vi "输入数据解析.vi"(0 "单个参数补充":dbl, 1 "从板号":dbl=1.0, 2 "主板二维码":string="BNET01", 3 "从板二维码":string="BNET01", 5 "主板引用":refnum<vi>, 7 "从板引用":refnum<vi>, 9 "主板选项":string="三级故障阀值", 11 "枚举":enum16{"主板", "从板"}(ring), 12 "快换":bool caption="快换写入") -> (4 "输出数组":dbl[][](array[numeric]), 6 "数组长度":dbl[](array[numeric]), 8 "循环次数":i32, 10 "命令":u32, 14 "名称":string[](array[string]), 15 "命令序号":u32[](array[numeric]))   [LabVIEW 2013] (continued)
                    n679 = call "输入分辨率计算-EV05.vi"("1字节?"=TRUE, "数值"=w1608, "偏移量"=0.0, "分辨率"=1.0) -> ("高字节1"=w1611:dbl)  [unwired: 1 in, 6 out]
                  }
                  frame Enabled {
                  }
                }
                n680 = Build Array(w1607) -> (w1606:i32[])
              }
              frame 12 {
                # "SOC过高"
                n681 = Unbundle By Name(w1619) -> ("SOC过高"=w1618:dbl)
                n682 = call "输入分辨率计算-EV05.vi"("1字节?"=FALSE, "数值"=w1618, "偏移量"=0.0, "分辨率"=0.1) -> ("低字节"=w1620:dbl, "高字节1"=w1621:dbl)  [unwired: 1 in, 5 out]
                n683 = call "二进制解析-8.6.vi"("索引"=4, "数值"=w1621) -> ("低位子数组"=w1624:i32[])  [unwired: 3 out]
                n684 = call "二进制解析-8.6.vi"("索引"=4, "数值"=w1620) -> ("低位子数组"=w1616:i32[], "高位子数组"=w1623:i32[])  [unwired: 2 out]
                n685 = Insert Into Array(array=w1624, new element=w1623) -> (w1622:i32[])  [unwired: 1 in]
                n686 = call "数值二进制转十进制-8.6.vi"("子数组"=w1622) -> ("十进制数值"=w1617:i32)  [unwired: 4 out]
                n687 = disable-structure shown="启用" {
                  disable-tunnel: w1617 -> [w1632 _]
                  disable-tunnel: [w1632 255 ("高字节1")] -> w1615
                  disable-tunnel: [w1631 i32[] [] ("低位子数组 20")] -> _
                  disable-tunnel: w1616 -> [w1631 _]
                  frame Disabled {
                  }
                  frame Enabled {
                  }
                }
                n688 = Build Array(w1615, w1615) -> (w1628:i32[])
              }
              frame 13 {
                # "SOC过低"
                n689 = Unbundle By Name(w1641) -> ("SOC过低"=w1640:dbl)
                n690 = call "输入分辨率计算-EV05.vi"("1字节?"=FALSE, "数值"=w1640, "偏移量"=0.0, "分辨率"=0.1) -> ("低字节"=w1638:dbl, "高字节1"=w1639:dbl)  [unwired: 1 in, 5 out]
                n691 = call "二进制解析-8.6.vi"("索引"=4, "数值"=w1639) -> ("低位子数组"=w1636:i32[])  [unwired: 3 out]
                n692 = disable-structure shown="启用" {
                  disable-tunnel: w1638 -> [w1648 _]
                  disable-tunnel: [w1648 255 ("高字节1")] -> w1637
                  disable-tunnel: w1636 -> [w1647 _]
                  disable-tunnel: [_ 255 ("高字节1")] -> w1635
                  frame Disabled {
                    (unwired) i32[] [] ("低位子数组 4")
                  }
                  frame Enabled {
                  }
                }
                n693 = Build Array(w1635, w1637) -> (w1644:i32[])
              }
              frame 14 {
                # "内阻过大"
                n694 = disable-structure shown="启用" {
                  disable-tunnel: w1653 -> [w1658 _]
                  disable-tunnel: [w1654 255 ("高字节1")] -> w1651
                  frame Disabled {
                    n695 = Unbundle By Name(w1658) -> ("内阻过大"=w1657:dbl)
                    n696 = call "输入分辨率计算-EV05.vi"("1字节?"=TRUE, "数值"=w1657, "分辨率"=0.1) -> ("高字节1"=w1654:dbl)  [unwired: 2 in, 6 out]
                  }
                  frame Enabled {
                  }
                }
                n697 = Build Array(w1651) -> (w1652:i32[])
              }
              frame 15 {
                # "极柱温度过高"
                n698 = disable-structure shown="启用" {
                  disable-tunnel: w1662 -> [w1668 _]
                  disable-tunnel: [w1664 255 ("高字节1")] -> w1660
                  frame Disabled {
                    n699 = Unbundle By Name(w1668) -> ("极柱温度过高"=w1667:dbl)
                    n700 = call "输入分辨率计算-EV05.vi"("1字节?"=TRUE, "数值"=w1667, "偏移量"=-40.0, "分辨率"=1.0) -> ("高字节1"=w1664:dbl)  [unwired: 1 in, 6 out]
                  }
                  frame Enabled {
                  }
                }
                n701 = Build Array(w1660) -> (w1661:i32[])
              }
              frame 16 {
                # "SOH过低"
                n702 = disable-structure shown="启用" {
                  disable-tunnel: [w1685 w1693] -> w1672
                  disable-tunnel: w1671 -> [w1682 _]
                  disable-tunnel: [w1674 w1693] -> w1670
                  frame Disabled {
                    n703 = Unbundle By Name(w1682) -> ("SOH过低"=w1681:dbl)
                    n704 = call "输入分辨率计算-EV05.vi"("1字节?"=FALSE, "数值"=w1681, "偏移量"=0.0, "分辨率"=0.1) -> ("低字节"=w1683:dbl, "高字节1"=w1684:dbl)  [unwired: 1 in, 5 out]
                    n705 = call "二进制解析-8.6.vi"("索引"=4, "数值"=w1684) -> ("低位子数组"=w1687:i32[])  [unwired: 3 out]
                    n706 = call "二进制解析-8.6.vi"("索引"=4, "数值"=w1683) -> ("低位子数组"=w1676:i32[], "高位子数组"=w1686:i32[])  [unwired: 2 out]
                    n707 = call "二进制解析-8.6.vi"("索引"=4, "数值"=0) -> ("低位子数组"=w1677:i32[])  [unwired: 3 out]
                    n708 = Insert Into Array(array=w1687, new element=w1686) -> (w1680:i32[])  [unwired: 1 in]
                    n709 = Insert Into Array(array=w1676, new element=w1677) -> (w1675:i32[])  [unwired: 1 in]
                    n710 = call "数值二进制转十进制-8.6.vi"("子数组"=w1680) -> ("十进制数值"=w1685:i32)  [unwired: 4 out]
                    n711 = call "数值二进制转十进制-8.6.vi"("子数组"=w1675) -> ("十进制数值"=w1674:i32)  [unwired: 4 out]
                  }
                  frame Enabled {
                    w1693 = 255 ("高字节1")
                  }
                }
                n712 = Build Array(w1672, w1670) -> (w1673:i32[])
              }
            }
            n713 = Insert Into Array(array=w1477, new element=w1478) -> (w1476:dbl[])  [unwired: 1 in]
          }
          n714 = Build Array(w1473) -> (w1472:dbl[][])
          n715 = Build Array("一级故障阀值") -> (w1463:string[])
        }
        frame "总电压过低(2)" {
          n716 = Unbundle By Name(w1699) -> ("一级故障 2"=w1700:refnum<vi>)
          n717 = property class="Clust (严格)"(reference=w1700) -> ("Value"=w1698:T4)  [unwired: 1 in, 2 out]
          n718 = for {
            N: 17 -> [_]
            tunnel: w1698 -> [w1710]
            shift-right: [w1707] -> w1704
            shift-left: dbl[] [] -> [w1708]
            i -> [w1711]
            n719 = case shown="13" w1711 {
              tunnel: w1710 -> [w1712 w1723 w1734 w1744 w1754 w1764 w1776 w1788 w1800 w1812 w1824 w1836 w1850 w1872 w1884 w1893 w1902]
              tunnel: [w1713 w1724 w1735 w1745 w1755 w1766 w1778 w1790 w1802 w1814 w1826 w1837 w1859 w1875 w1883 w1892 w1904] -> w1709
              frame 0, Default {
                # "总电压过高"
                n720 = disable-structure shown="启用" {
                  disable-tunnel: [w1719 w1722] -> w1715
                  disable-tunnel: [w1718 w1722] -> w1714
                  disable-tunnel: w1712 -> [w1717 _]
                  frame Disabled {
                    n721 = Unbundle By Name(w1717) -> ("总电压过高"=w1716:dbl)
                    n722 = call "输入分辨率计算-EV05.vi"("1字节?"=FALSE, "数值"=w1716, "分辨率"=0.1) -> ("低字节"=w1719:dbl, "高字节1"=w1718:dbl)  [unwired: 2 in, 5 out]
                  }
                  frame Enabled {
                    w1722 = 255 ("高字节1")
                  }
                }
                n723 = Build Array(w1714, w1715) -> (w1713:i32[])
              }
              frame 1 {
                # "总电压过低"
                n724 = disable-structure shown="启用" {
                  disable-tunnel: [w1730 w1733] -> w1726
                  disable-tunnel: [w1729 w1733] -> w1725
                  disable-tunnel: w1723 -> [w1728 _]
                  frame Enabled {
                    n725 = Unbundle By Name(w1728) -> ("总电压过低"=w1727:dbl)
                    n726 = call "输入分辨率计算-EV05.vi"("1字节?"=FALSE, "数值"=w1727, "分辨率"=0.1) -> ("低字节"=w1730:dbl, "高字节1"=w1729:dbl)  [unwired: 2 in, 5 out]
                  }
                  frame Disabled {
                    w1733 = 255 ("高字节1")
                  }
                }
                n727 = Build Array(w1725, w1726) -> (w1724:dbl[])
              }
              frame 2 {
                # "温度过高"
                n728 = disable-structure shown="启用" {
                  disable-tunnel: [w1740 255 ("高字节1")] -> w1736
                  disable-tunnel: w1734 -> [w1738 _]
                  frame Disabled {
                    n729 = Unbundle By Name(w1738) -> ("温度过高"=w1737:dbl)
                    n730 = call "输入分辨率计算-EV05.vi"("1字节?"=TRUE, "数值"=w1737, "偏移量"=-40.0, "分辨率"=1.0) -> ("高字节1"=w1740:dbl)  [unwired: 1 in, 6 out]
                  }
                  frame Enabled {
                  }
                }
                n731 = Build Array(w1736) -> (w1735:i32[])
              }
              frame 3 {
                # "温度过低"
                n732 = disable-structure shown="启用" {
                  disable-tunnel: [w1750 255 ("高字节1")] -> w1746
                  disable-tunnel: w1744 -> [w1748 _]
                  frame Disabled {
                    n733 = Unbundle By Name(w1748) -> ("温度过低"=w1747:dbl)
                    n734 = call "输入分辨率计算-EV05.vi"("1字节?"=TRUE, "数值"=w1747, "偏移量"=-40.0, "分辨率"=1.0) -> ("高字节1"=w1750:dbl)  [unwired: 1 in, 6 out]
                  }
                  frame Enabled {
                  }
                }
                n735 = Build Array(w1746) -> (w1745:i32[])
              }
              frame 4 {
                # "整组温度不均衡"
                n736 = disable-structure shown="启用" {
                  disable-tunnel: [w1760 255 ("高字节1")] -> w1756
                  disable-tunnel: w1754 -> [w1758 _]
                  frame Disabled {
                    n737 = Unbundle By Name(w1758) -> ("整组温度不均衡"=w1757:dbl)
                    n738 = call "输入分辨率计算-EV05.vi"("1字节?"=TRUE, "数值"=w1757, "偏移量"=0.0, "分辨率"=1.0) -> ("高字节1"=w1760:dbl)  [unwired: 1 in, 6 out]
                  }
                  frame Enabled {
                  }
                }
                n739 = Build Array(w1756) -> (w1755:i32[])
              }
              frame 5 {
                # "单组电压不均衡"
                n740 = disable-structure shown="启用" {
                  disable-tunnel: [w1772 w1775] -> w1767
                  disable-tunnel: [w1770 w1775] -> w1765
                  disable-tunnel: w1764 -> [w1769 _]
                  frame Disabled {
                    n741 = Unbundle By Name(w1769) -> ("单组电压不均衡"=w1768:dbl)
                    n742 = call "输入分辨率计算-EV05.vi"("1字节?"=FALSE, "数值"=w1768, "偏移量"=0.0, "分辨率"=0.001) -> ("低字节"=w1770:dbl, "高字节1"=w1772:dbl)  [unwired: 1 in, 5 out]
                  }
                  frame Enabled {
                    w1775 = 255 ("高字节1")
                  }
                }
                n743 = Build Array(w1767, w1765) -> (w1766:i32[])
              }
              frame 6 {
                # "整组电压不均衡"
                n744 = disable-structure shown="启用" {
                  disable-tunnel: [w1784 w1787] -> w1779
                  disable-tunnel: [w1782 w1787] -> w1777
                  disable-tunnel: w1776 -> [w1781 _]
                  frame Disabled {
                    n745 = Unbundle By Name(w1781) -> ("整组电压不均衡"=w1780:dbl)
                    n746 = call "输入分辨率计算-EV05.vi"("1字节?"=FALSE, "数值"=w1780, "偏移量"=0.0, "分辨率"=0.001) -> ("低字节"=w1782:dbl, "高字节1"=w1784:dbl)  [unwired: 1 in, 5 out]
                  }
                  frame Enabled {
                    w1787 = 255 ("高字节1")
                  }
                }
                n747 = Build Array(w1779, w1777) -> (w1778:i32[])
              }
              frame 7 {
                # "单体电压过高"
                n748 = disable-structure shown="启用" {
                  disable-tunnel: [w1796 w1799] -> w1791
                  disable-tunnel: [w1794 w1799] -> w1789
                  disable-tunnel: w1788 -> [w1793 _]
                  frame Disabled {
                    n749 = Unbundle By Name(w1793) -> ("单体电压过高"=w1792:dbl)
                    n750 = call "输入分辨率计算-EV05.vi"("1字节?"=FALSE, "数值"=w1792, "偏移量"=0.0, "分辨率"=0.001) -> ("低字节"=w1794:dbl, "高字节1"=w1796:dbl)  [unwired: 1 in, 5 out]
                  }
                  frame Enabled {
                    w1799 = 255 ("高字节1")
                  }
                }
                n751 = Build Array(w1791, w1789) -> (w1790:i32[])
              }
              frame 8 {
                # "单体电压过低"
                n752 = disable-structure shown="启用" {
                  disable-tunnel: [w1808 w1811] -> w1803
                  disable-tunnel: [w1806 w1811] -> w1801
                  disable-tunnel: w1800 -> [w1805 _]
                  frame Disabled {
                    n753 = Unbundle By Name(w1805) -> ("单体电压过低"=w1804:dbl)
                    n754 = call "输入分辨率计算-EV05.vi"("1字节?"=FALSE, "数值"=w1804, "偏移量"=0.0, "分辨率"=0.001) -> ("低字节"=w1806:dbl, "高字节1"=w1808:dbl)  [unwired: 1 in, 5 out]
                  }
                  frame Enabled {
                    w1811 = 255 ("高字节1")
                  }
                }
                n755 = Build Array(w1803, w1801) -> (w1802:i32[])
              }
              frame 9 {
                # "充电电流过高"
                n756 = disable-structure shown="启用" {
                  disable-tunnel: [w1820 w1823] -> w1815
                  disable-tunnel: [w1818 w1823] -> w1813
                  disable-tunnel: w1812 -> [w1817 _]
                  frame Disabled {
                    n757 = Unbundle By Name(w1817) -> ("充电电流过高"=w1816:dbl)
                    n758 = call "输入分辨率计算-EV05.vi"("1字节?"=FALSE, "数值"=w1816, "偏移量"=-3000.0, "分辨率"=0.1) -> ("低字节"=w1818:dbl, "高字节1"=w1820:dbl)  [unwired: 1 in, 5 out]
                  }
                  frame Enabled {
                    w1823 = 255 ("高字节1")
                  }
                }
                n759 = Build Array(w1815, w1813) -> (w1814:i32[])
              }
              frame 10 {
                # "放电电流过高"
                n760 = disable-structure shown="启用" {
                  disable-tunnel: [w1832 w1835] -> w1827
                  disable-tunnel: [w1830 w1835] -> w1825
                  disable-tunnel: w1824 -> [w1829 _]
                  frame Disabled {
                    n761 = Unbundle By Name(w1829) -> ("放电电流过高"=w1828:dbl)
                    n762 = call "输入分辨率计算-EV05.vi"("1字节?"=FALSE, "数值"=w1828, "偏移量"=-3000.0, "分辨率"=0.1) -> ("低字节"=w1830:dbl, "高字节1"=w1832:dbl)  [unwired: 1 in, 5 out]
                  }
                  frame Enabled {
                    w1835 = 255 ("高字节1")
                  }
                }
                n763 = Build Array(w1827, w1825) -> (w1826:i32[])
              }
              frame 11 {
                # "单组温度不均衡"
                n764 = disable-structure shown="启用" {
                  disable-tunnel: [w1842 255 ("高字节1")] -> w1838
                  disable-tunnel: w1836 -> [w1840 _]
                  frame Disabled {
                    n765 = Unbundle By Name(w1840) -> ("单组温度不均衡"=w1839:dbl)
                    n766 = call "输入分辨率计算-EV05.vi"("1字节?"=TRUE, "数值"=w1839, "偏移量"=0.0, "分辨率"=1.0) -> ("高字节1"=w1842:dbl)  [unwired: 1 in, 6 out]
                  }
                  frame Enabled {
                  }
                }
                n767 = Build Array(w1838) -> (w1837:i32[])
              }
              frame 12 {
                # "SOC过高"
                n768 = Unbundle By Name(w1850) -> ("SOC过高"=w1849:dbl)
                n769 = call "输入分辨率计算-EV05.vi"("1字节?"=FALSE, "数值"=w1849, "偏移量"=0.0, "分辨率"=0.1) -> ("低字节"=w1851:dbl, "高字节1"=w1852:dbl)  [unwired: 1 in, 5 out]
                n770 = call "二进制解析-8.6.vi"("索引"=4, "数值"=w1852) -> ("低位子数组"=w1855:i32[])  [unwired: 3 out]
                n771 = call "二进制解析-8.6.vi"("索引"=4, "数值"=w1851) -> ("低位子数组"=w1847:i32[], "高位子数组"=w1854:i32[])  [unwired: 2 out]
                n772 = Insert Into Array(array=w1855, new element=w1854) -> (w1853:i32[])  [unwired: 1 in]
                n773 = call "数值二进制转十进制-8.6.vi"("子数组"=w1853) -> ("十进制数值"=w1848:i32)  [unwired: 4 out]
                n774 = disable-structure shown="启用" {
                  disable-tunnel: w1848 -> [w1863 _]
                  disable-tunnel: [w1863 255 ("高字节1")] -> w1846
                  disable-tunnel: [w1862 i32[] [] ("低位子数组 20")] -> _
                  disable-tunnel: w1847 -> [w1862 _]
                  frame Disabled {
                  }
                  frame Enabled {
                  }
                }
                n775 = Build Array(w1846, w1846) -> (w1859:i32[])
              }
              frame 13 {
                # "SOC过低"
                n776 = Unbundle By Name(w1872) -> ("SOC过低"=w1871:dbl)
                n777 = call "输入分辨率计算-EV05.vi"("1字节?"=FALSE, "数值"=w1871, "偏移量"=0.0, "分辨率"=0.1) -> ("低字节"=w1869:dbl, "高字节1"=w1870:dbl)  [unwired: 1 in, 5 out]
                n778 = call "二进制解析-8.6.vi"("索引"=4, "数值"=w1870) -> ("低位子数组"=w1867:i32[])  [unwired: 3 out]
                n779 = disable-structure shown="启用" {
                  disable-tunnel: w1869 -> [w1879 _]
                  disable-tunnel: [w1879 255 ("高字节1")] -> w1868
                  disable-tunnel: w1867 -> [w1878 _]
                  disable-tunnel: [_ 255 ("高字节1")] -> w1866
                  frame Disabled {
                    (unwired) i32[] [] ("低位子数组 4")
                  }
                  frame Enabled {
                  }
                }
                n780 = Build Array(w1866, w1868) -> (w1875:i32[])
              }
              frame 14 {
                # "内阻过大"
                n781 = disable-structure shown="启用" {
                  disable-tunnel: w1884 -> [w1889 _]
                  disable-tunnel: [w1885 255 ("高字节1")] -> w1882
                  frame Disabled {
                    n782 = Unbundle By Name(w1889) -> ("内阻过大"=w1888:dbl)
                    n783 = call "输入分辨率计算-EV05.vi"("1字节?"=TRUE, "数值"=w1888, "分辨率"=0.1) -> ("高字节1"=w1885:dbl)  [unwired: 2 in, 6 out]
                  }
                  frame Enabled {
                  }
                }
                n784 = Build Array(w1882) -> (w1883:i32[])
              }
              frame 15 {
                # "极柱温度过高"
                n785 = disable-structure shown="启用" {
                  disable-tunnel: w1893 -> [w1899 _]
                  disable-tunnel: [w1895 255 ("高字节1")] -> w1891
                  frame Disabled {
                    n786 = Unbundle By Name(w1899) -> ("极柱温度过高"=w1898:dbl)
                    n787 = call "输入分辨率计算-EV05.vi"("1字节?"=TRUE, "数值"=w1898, "偏移量"=-40.0, "分辨率"=1.0) -> ("高字节1"=w1895:dbl)  [unwired: 1 in, 6 out]
                  }
                  frame Enabled {
                  }
                }
                n788 = Build Array(w1891) -> (w1892:i32[])
              }
              frame 16 {
                # "SOH过低"
                n789 = disable-structure shown="启用" {
                  disable-tunnel: [w1916 w1924] -> w1903
                  disable-tunnel: w1902 -> [w1913 _]
                  disable-tunnel: [w1905 w1924] -> w1901
                  frame Disabled {
                    n790 = Unbundle By Name(w1913) -> ("SOH过低"=w1912:dbl)
                    n791 = call "输入分辨率计算-EV05.vi"("1字节?"=FALSE, "数值"=w1912, "偏移量"=0.0, "分辨率"=0.1) -> ("低字节"=w1914:dbl, "高字节1"=w1915:dbl)  [unwired: 1 in, 5 out]
                    n792 = call "二进制解析-8.6.vi"("索引"=4, "数值"=w1915) -> ("低位子数组"=w1918:i32[])  [unwired: 3 out]
                    n793 = call "二进制解析-8.6.vi"("索引"=4, "数值"=w1914) -> ("低位子数组"=w1907:i32[], "高位子数组"=w1917:i32[])  [unwired: 2 out]
                    n794 = call "二进制解析-8.6.vi"("索引"=4, "数值"=0) -> ("低位子数组"=w1908:i32[])  [unwired: 3 out]
                    n795 = Insert Into Array(array=w1918, new element=w1917) -> (w1911:i32[])  [unwired: 1 in]
                    n796 = Insert Into Array(array=w1907, new element=w1908) -> (w1906:i32[])  [unwired: 1 in]
                    n797 = call "数值二进制转十进制-8.6.vi"("子数组"=w1911) -> ("十进制数值"=w1916:i32)  [unwired: 4 out]
                    n798 = call "数值二进制转十进制-8.6.vi"("子数组"=w1906) -> ("十进制数值"=w1905:i32)  [unwired: 4 out]
                  }
                  frame Enabled {
                    w1924 = 255 ("高字节1")
                  }
                }
                n799 = Build Array(w1903, w1901) -> (w1904:i32[])
              }
            }
            n800 = Insert Into Array(array=w1708, new element=w1709) -> (w1707:dbl[])  [unwired: 1 in]
          }
          n801 = Build Array(w1704) -> (w1703:dbl[][])
          n802 = Build Array("二级故障阀值") -> (w1694:string[])
        }
        frame "总电压过低(3)" {
          n803 = Unbundle By Name(w1930) -> ("一级故障 3"=w1931:refnum<vi>)
          n804 = property class="Clust (严格)"(reference=w1931) -> ("Value"=w1929:T4)  [unwired: 1 in, 2 out]
          n805 = for {
            N: 17 -> [_]
            tunnel: w1929 -> [w1941]
            shift-right: [w1938] -> w1935
            shift-left: dbl[] [] -> [w1939]
            i -> [w1942]
            n806 = case shown="13" w1942 {
              tunnel: w1941 -> [w1943 w1954 w1965 w1975 w1985 w1995 w2007 w2019 w2031 w2043 w2055 w2067 w2081 w2103 w2115 w2124 w2133]
              tunnel: [w1944 w1955 w1966 w1976 w1986 w1997 w2009 w2021 w2033 w2045 w2057 w2068 w2090 w2106 w2114 w2123 w2135] -> w1940
              frame 0, Default {
                # "总电压过高"
                n807 = disable-structure shown="启用" {
                  disable-tunnel: [w1950 w1953] -> w1946
                  disable-tunnel: [w1949 w1953] -> w1945
                  disable-tunnel: w1943 -> [w1948 _]
                  frame Disabled {
                    n808 = Unbundle By Name(w1948) -> ("总电压过高"=w1947:dbl)
                    n809 = call "输入分辨率计算-EV05.vi"("1字节?"=FALSE, "数值"=w1947, "分辨率"=0.1) -> ("低字节"=w1950:dbl, "高字节1"=w1949:dbl)  [unwired: 2 in, 5 out]
                  }
                  frame Enabled {
                    w1953 = 255 ("高字节1")
                  }
                }
                n810 = Build Array(w1945, w1946) -> (w1944:i32[])
              }
              frame 1 {
                # "总电压过低"
                n811 = disable-structure shown="启用" {
                  disable-tunnel: [w1961 w1964] -> w1957
                  disable-tunnel: [w1960 w1964] -> w1956
                  disable-tunnel: w1954 -> [w1959 _]
                  frame Enabled {
                    n812 = Unbundle By Name(w1959) -> ("总电压过低"=w1958:dbl)
                    n813 = call "输入分辨率计算-EV05.vi"("1字节?"=FALSE, "数值"=w1958, "分辨率"=0.1) -> ("低字节"=w1961:dbl, "高字节1"=w1960:dbl)  [unwired: 2 in, 5 out]
                  }
                  frame Disabled {
                    w1964 = 255 ("高字节1")
                  }
                }
                n814 = Build Array(w1956, w1957) -> (w1955:dbl[])
              }
              frame 2 {
                # "温度过高"
                n815 = disable-structure shown="启用" {
                  disable-tunnel: [w1971 255 ("高字节1")] -> w1967
                  disable-tunnel: w1965 -> [w1969 _]
                  frame Disabled {
                    n816 = Unbundle By Name(w1969) -> ("温度过高"=w1968:dbl)
                    n817 = call "输入分辨率计算-EV05.vi"("1字节?"=TRUE, "数值"=w1968, "偏移量"=-40.0, "分辨率"=1.0) -> ("高字节1"=w1971:dbl)  [unwired: 1 in, 6 out]
                  }
                  frame Enabled {
                  }
                }
                n818 = Build Array(w1967) -> (w1966:i32[])
              }
              frame 3 {
                # "温度过低"
                n819 = disable-structure shown="启用" {
                  disable-tunnel: [w1981 255 ("高字节1")] -> w1977
                  disable-tunnel: w1975 -> [w1979 _]
                  frame Disabled {
                    n820 = Unbundle By Name(w1979) -> ("温度过低"=w1978:dbl)
                    n821 = call "输入分辨率计算-EV05.vi"("1字节?"=TRUE, "数值"=w1978, "偏移量"=-40.0, "分辨率"=1.0) -> ("高字节1"=w1981:dbl)  [unwired: 1 in, 6 out]
                  }
                  frame Enabled {
                  }
                }
                n822 = Build Array(w1977) -> (w1976:i32[])
              }
              frame 4 {
                # "整组温度不均衡"
                n823 = disable-structure shown="启用" {
                  disable-tunnel: [w1991 255 ("高字节1")] -> w1987
                  disable-tunnel: w1985 -> [w1989 _]
                  frame Disabled {
                    n824 = Unbundle By Name(w1989) -> ("整组温度不均衡"=w1988:dbl)
                    n825 = call "输入分辨率计算-EV05.vi"("1字节?"=TRUE, "数值"=w1988, "偏移量"=0.0, "分辨率"=1.0) -> ("高字节1"=w1991:dbl)  [unwired: 1 in, 6 out]
                  }
                  frame Enabled {
                  }
                }
                n826 = Build Array(w1987) -> (w1986:i32[])
              }
              frame 5 {
                # "单组电压不均衡"
                n827 = disable-structure shown="启用" {
                  disable-tunnel: [w2003 w2006] -> w1998
                  disable-tunnel: [w2001 w2006] -> w1996
                  disable-tunnel: w1995 -> [w2000 _]
                  frame Disabled {
                    n828 = Unbundle By Name(w2000) -> ("单组电压不均衡"=w1999:dbl)
                    n829 = call "输入分辨率计算-EV05.vi"("1字节?"=FALSE, "数值"=w1999, "偏移量"=0.0, "分辨率"=0.001) -> ("低字节"=w2001:dbl, "高字节1"=w2003:dbl)  [unwired: 1 in, 5 out]
                  }
                  frame Enabled {
                    w2006 = 255 ("高字节1")
                  }
                }
                n830 = Build Array(w1998, w1996) -> (w1997:i32[])
              }
              frame 6 {
                # "整组电压不均衡"
                n831 = disable-structure shown="启用" {
                  disable-tunnel: [w2015 w2018] -> w2010
                  disable-tunnel: [w2013 w2018] -> w2008
                  disable-tunnel: w2007 -> [w2012 _]
                  frame Disabled {
                    n832 = Unbundle By Name(w2012) -> ("整组电压不均衡"=w2011:dbl)
                    n833 = call "输入分辨率计算-EV05.vi"("1字节?"=FALSE, "数值"=w2011, "偏移量"=0.0, "分辨率"=0.001) -> ("低字节"=w2013:dbl, "高字节1"=w2015:dbl)  [unwired: 1 in, 5 out]
                  }
                  frame Enabled {
                    w2018 = 255 ("高字节1")
                  }
                }
                n834 = Build Array(w2010, w2008) -> (w2009:i32[])
              }
              frame 7 {
                # "单体电压过高"
                n835 = disable-structure shown="启用" {
                  disable-tunnel: [w2027 w2030] -> w2022
                  disable-tunnel: [w2025 w2030] -> w2020
                  disable-tunnel: w2019 -> [w2024 _]
                  frame Disabled {
                    n836 = Unbundle By Name(w2024) -> ("单体电压过高"=w2023:dbl)
                    n837 = call "输入分辨率计算-EV05.vi"("1字节?"=FALSE, "数值"=w2023, "偏移量"=0.0, "分辨率"=0.001) -> ("低字节"=w2025:dbl, "高字节1"=w2027:dbl)  [unwired: 1 in, 5 out]
                  }
                  frame Enabled {
                    w2030 = 255 ("高字节1")
                  }
                }
                n838 = Build Array(w2022, w2020) -> (w2021:i32[])
              }
              frame 8 {
                # "单体电压过低"
                n839 = disable-structure shown="启用" {
                  disable-tunnel: [w2039 w2042] -> w2034
                  disable-tunnel: [w2037 w2042] -> w2032
                  disable-tunnel: w2031 -> [w2036 _]
                  frame Disabled {
                    n840 = Unbundle By Name(w2036) -> ("单体电压过低"=w2035:dbl)
                    n841 = call "输入分辨率计算-EV05.vi"("1字节?"=FALSE, "数值"=w2035, "偏移量"=0.0, "分辨率"=0.001) -> ("低字节"=w2037:dbl, "高字节1"=w2039:dbl)  [unwired: 1 in, 5 out]
                  }
                  frame Enabled {
                    w2042 = 255 ("高字节1")
                  }
                }
                n842 = Build Array(w2034, w2032) -> (w2033:i32[])
              }
              frame 9 {
                # "充电电流过高"
                n843 = disable-structure shown="启用" {
                  disable-tunnel: [w2051 w2054] -> w2046
                  disable-tunnel: [w2049 w2054] -> w2044
                  disable-tunnel: w2043 -> [w2048 _]
                  frame Disabled {
                    n844 = Unbundle By Name(w2048) -> ("充电电流过高"=w2047:dbl)
                    n845 = call "输入分辨率计算-EV05.vi"("1字节?"=FALSE, "数值"=w2047, "偏移量"=-3000.0, "分辨率"=0.1) -> ("低字节"=w2049:dbl, "高字节1"=w2051:dbl)  [unwired: 1 in, 5 out]
                  }
                  frame Enabled {
                    w2054 = 255 ("高字节1")
                  }
                }
                n846 = Build Array(w2046, w2044) -> (w2045:i32[])
              }
              frame 10 {
                # "放电电流过高"
                n847 = disable-structure shown="启用" {
                  disable-tunnel: [w2063 w2066] -> w2058
                  disable-tunnel: [w2061 w2066] -> w2056
                  disable-tunnel: w2055 -> [w2060 _]
                  frame Disabled {
                    n848 = Unbundle By Name(w2060) -> ("放电电流过高"=w2059:dbl)
                    n849 = call "输入分辨率计算-EV05.vi"("1字节?"=FALSE, "数值"=w2059, "偏移量"=-3000.0, "分辨率"=0.1) -> ("低字节"=w2061:dbl, "高字节1"=w2063:dbl)  [unwired: 1 in, 5 out]
                  }
                  frame Enabled {
                    w2066 = 255 ("高字节1")
                  }
                }
                n850 = Build Array(w2058, w2056) -> (w2057:i32[])
              }
              frame 11 {
                # "单组温度不均衡"
                n851 = disable-structure shown="启用" {
                  disable-tunnel: [w2073 255 ("高字节1")] -> w2069
                  disable-tunnel: w2067 -> [w2071 _]
                  frame Disabled {
                    n852 = Unbundle By Name(w2071) -> ("单组温度不均衡"=w2070:dbl)
                    n853 = call "输入分辨率计算-EV05.vi"("1字节?"=TRUE, "数值"=w2070, "偏移量"=0.0, "分辨率"=1.0) -> ("高字节1"=w2073:dbl)  [unwired: 1 in, 6 out]
                  }
                  frame Enabled {
                  }
                }
                n854 = Build Array(w2069) -> (w2068:i32[])
              }
              frame 12 {
                # "SOC过高"
                n855 = Unbundle By Name(w2081) -> ("SOC过高"=w2080:dbl)
                n856 = call "输入分辨率计算-EV05.vi"("1字节?"=FALSE, "数值"=w2080, "偏移量"=0.0, "分辨率"=0.1) -> ("低字节"=w2082:dbl, "高字节1"=w2083:dbl)  [unwired: 1 in, 5 out]
                n857 = call "二进制解析-8.6.vi"("索引"=4, "数值"=w2083) -> ("低位子数组"=w2086:i32[])  [unwired: 3 out]
                n858 = call "二进制解析-8.6.vi"("索引"=4, "数值"=w2082) -> ("低位子数组"=w2078:i32[], "高位子数组"=w2085:i32[])  [unwired: 2 out]
                n859 = Insert Into Array(array=w2086, new element=w2085) -> (w2084:i32[])  [unwired: 1 in]
                n860 = call "数值二进制转十进制-8.6.vi"("子数组"=w2084) -> ("十进制数值"=w2079:i32)  [unwired: 4 out]
                n861 = disable-structure shown="启用" {
                  disable-tunnel: w2079 -> [w2094 _]
                  disable-tunnel: [w2094 255 ("高字节1")] -> w2077
                  disable-tunnel: [w2093 i32[] [] ("低位子数组 20")] -> _
                  disable-tunnel: w2078 -> [w2093 _]
                  frame Disabled {
                  }
                  frame Enabled {
                  }
                }
                n862 = Build Array(w2077, w2077) -> (w2090:i32[])
              }
              frame 13 {
                # "SOC过低"
                n863 = Unbundle By Name(w2103) -> ("SOC过低"=w2102:dbl)
                n864 = call "输入分辨率计算-EV05.vi"("1字节?"=FALSE, "数值"=w2102, "偏移量"=0.0, "分辨率"=0.1) -> ("低字节"=w2100:dbl, "高字节1"=w2101:dbl)  [unwired: 1 in, 5 out]
                n865 = call "二进制解析-8.6.vi"("索引"=4, "数值"=w2101) -> ("低位子数组"=w2098:i32[])  [unwired: 3 out]
                n866 = disable-structure shown="启用" {
                  disable-tunnel: w2100 -> [w2110 _]
                  disable-tunnel: [w2110 255 ("高字节1")] -> w2099
                  disable-tunnel: w2098 -> [w2109 _]
                  disable-tunnel: [_ 255 ("高字节1")] -> w2097
                  frame Disabled {
                    (unwired) i32[] [] ("低位子数组 4")
                  }
                  frame Enabled {
                  }
                }
                n867 = Build Array(w2097, w2099) -> (w2106:i32[])
              }
              frame 14 {
                # "内阻过大"
                n868 = disable-structure shown="启用" {
                  disable-tunnel: w2115 -> [w2120 _]
                  disable-tunnel: [w2116 255 ("高字节1")] -> w2113
                  frame Disabled {
                    n869 = Unbundle By Name(w2120) -> ("内阻过大"=w2119:dbl)
                    n870 = call "输入分辨率计算-EV05.vi"("1字节?"=TRUE, "数值"=w2119, "分辨率"=0.1) -> ("高字节1"=w2116:dbl)  [unwired: 2 in, 6 out]
                  }
                  frame Enabled {
                  }
                }
                n871 = Build Array(w2113) -> (w2114:i32[])
              }
              frame 15 {
                # "极柱温度过高"
                n872 = disable-structure shown="启用" {
                  disable-tunnel: w2124 -> [w2130 _]
                  disable-tunnel: [w2126 255 ("高字节1")] -> w2122
                  frame Disabled {
                    n873 = Unbundle By Name(w2130) -> ("极柱温度过高"=w2129:dbl)
                    n874 = call "输入分辨率计算-EV05.vi"("1字节?"=TRUE, "数值"=w2129, "偏移量"=-40.0, "分辨率"=1.0) -> ("高字节1"=w2126:dbl)  [unwired: 1 in, 6 out]
                  }
                  frame Enabled {
                  }
                }
                n875 = Build Array(w2122) -> (w2123:i32[])
              }
              frame 16 {
                # "SOH过低"
                n876 = disable-structure shown="启用" {
                  disable-tunnel: [w2147 w2155] -> w2134
                  disable-tunnel: w2133 -> [w2144 _]
                  disable-tunnel: [w2136 w2155] -> w2132
                  frame Disabled {
                    n877 = Unbundle By Name(w2144) -> ("SOH过低"=w2143:dbl)
                    n878 = call "输入分辨率计算-EV05.vi"("1字节?"=FALSE, "数值"=w2143, "偏移量"=0.0, "分辨率"=0.1) -> ("低字节"=w2145:dbl, "高字节1"=w2146:dbl)  [unwired: 1 in, 5 out]
                    n879 = call "二进制解析-8.6.vi"("索引"=4, "数值"=w2146) -> ("低位子数组"=w2149:i32[])  [unwired: 3 out]
                    n880 = call "二进制解析-8.6.vi"("索引"=4, "数值"=w2145) -> ("低位子数组"=w2138:i32[], "高位子数组"=w2148:i32[])  [unwired: 2 out]
                    n881 = call "二进制解析-8.6.vi"("索引"=4, "数值"=0) -> ("低位子数组"=w2139:i32[])  [unwired: 3 out]
                    n882 = Insert Into Array(array=w2149, new element=w2148) -> (w2142:i32[])  [unwired: 1 in]
                    n883 = Insert Into Array(array=w2138, new element=w2139) -> (w2137:i32[])  [unwired: 1 in]
                    n884 = call "数值二进制转十进制-8.6.vi"("子数组"=w2142) -> ("十进制数值"=w2147:i32)  [unwired: 4 out]
                    n885 = call "数值二进制转十进制-8.6.vi"("子数组"=w2137) -> ("十进制数值"=w2136:i32)  [unwired: 4 out]
                  }
                  frame Enabled {
                    w2155 = 255 ("高字节1")
                  }
                }
                n886 = Build Array(w2134, w2132) -> (w2135:i32[])
              }
            }
            n887 = Insert Into Array(array=w1939, new element=w1940) -> (w1938:dbl[])  [unwired: 1 in]
          }
          n888 = Build Array(w1935) -> (w1934:dbl[][])
          n889 = Build Array("三级故障阀值") -> (w1925:string[])
        }
        frame "总电压过高(2)" {
          n890 = Unbundle By Name(w2161) -> ("一级故障 2"=w2162:refnum<vi>)
          n891 = property class="Clust (严格)"(reference=w2162) -> ("Value"=w2160:T4)  [unwired: 1 in, 2 out]
          n892 = for {
            N: 17 -> [_]
            tunnel: w2160 -> [w2172]
            shift-right: [w2169] -> w2166
            shift-left: dbl[] [] -> [w2170]
            i -> [w2173]
            n893 = case shown="13" w2173 {
              tunnel: w2172 -> [w2174 w2185 w2196 w2206 w2216 w2226 w2238 w2250 w2262 w2274 w2286 w2298 w2312 w2334 w2346 w2355 w2364]
              tunnel: [w2175 w2186 w2197 w2207 w2217 w2228 w2240 w2252 w2264 w2276 w2288 w2299 w2321 w2337 w2345 w2354 w2366] -> w2171
              frame 0, Default {
                # "总电压过高"
                n894 = disable-structure shown="启用" {
                  disable-tunnel: [w2181 w2184] -> w2177
                  disable-tunnel: [w2180 w2184] -> w2176
                  disable-tunnel: w2174 -> [w2179 _]
                  frame Enabled {
                    n895 = Unbundle By Name(w2179) -> ("总电压过高"=w2178:dbl)
                    n896 = call "输入分辨率计算-EV05.vi"("1字节?"=FALSE, "数值"=w2178, "分辨率"=0.1) -> ("低字节"=w2181:dbl, "高字节1"=w2180:dbl)  [unwired: 2 in, 5 out]
                  }
                  frame Disabled {
                    w2184 = 255 ("高字节1")
                  }
                }
                n897 = Build Array(w2176, w2177) -> (w2175:dbl[])
              }
              frame 1 {
                # "总电压过低"
                n898 = disable-structure shown="启用" {
                  disable-tunnel: [w2192 w2195] -> w2188
                  disable-tunnel: [w2191 w2195] -> w2187
                  disable-tunnel: w2185 -> [w2190 _]
                  frame Disabled {
                    n899 = Unbundle By Name(w2190) -> ("总电压过低"=w2189:dbl)
                    n900 = call "输入分辨率计算-EV05.vi"("1字节?"=FALSE, "数值"=w2189, "分辨率"=0.1) -> ("低字节"=w2192:dbl, "高字节1"=w2191:dbl)  [unwired: 2 in, 5 out]
                  }
                  frame Enabled {
                    w2195 = 255 ("高字节1")
                  }
                }
                n901 = Build Array(w2187, w2188) -> (w2186:i32[])
              }
              frame 2 {
                # "温度过高"
                n902 = disable-structure shown="启用" {
                  disable-tunnel: [w2202 255 ("高字节1")] -> w2198
                  disable-tunnel: w2196 -> [w2200 _]
                  frame Disabled {
                    n903 = Unbundle By Name(w2200) -> ("温度过高"=w2199:dbl)
                    n904 = call "输入分辨率计算-EV05.vi"("1字节?"=TRUE, "数值"=w2199, "偏移量"=-40.0, "分辨率"=1.0) -> ("高字节1"=w2202:dbl)  [unwired: 1 in, 6 out]
                  }
                  frame Enabled {
                  }
                }
                n905 = Build Array(w2198) -> (w2197:i32[])
              }
              frame 3 {
                # "温度过低"
                n906 = disable-structure shown="启用" {
                  disable-tunnel: [w2212 255 ("高字节1")] -> w2208
                  disable-tunnel: w2206 -> [w2210 _]
                  frame Disabled {
                    n907 = Unbundle By Name(w2210) -> ("温度过低"=w2209:dbl)
                    n908 = call "输入分辨率计算-EV05.vi"("1字节?"=TRUE, "数值"=w2209, "偏移量"=-40.0, "分辨率"=1.0) -> ("高字节1"=w2212:dbl)  [unwired: 1 in, 6 out]
                  }
                  frame Enabled {
                  }
                }
                n909 = Build Array(w2208) -> (w2207:i32[])
              }
              frame 4 {
                # "整组温度不均衡"
                n910 = disable-structure shown="启用" {
                  disable-tunnel: [w2222 255 ("高字节1")] -> w2218
                  disable-tunnel: w2216 -> [w2220 _]
                  frame Disabled {
                    n911 = Unbundle By Name(w2220) -> ("整组温度不均衡"=w2219:dbl)
                    n912 = call "输入分辨率计算-EV05.vi"("1字节?"=TRUE, "数值"=w2219, "偏移量"=0.0, "分辨率"=1.0) -> ("高字节1"=w2222:dbl)  [unwired: 1 in, 6 out]
                  }
                  frame Enabled {
                  }
                }
                n913 = Build Array(w2218) -> (w2217:i32[])
              }
              frame 5 {
                # "单组电压不均衡"
                n914 = disable-structure shown="启用" {
                  disable-tunnel: [w2234 w2237] -> w2229
                  disable-tunnel: [w2232 w2237] -> w2227
                  disable-tunnel: w2226 -> [w2231 _]
                  frame Disabled {
                    n915 = Unbundle By Name(w2231) -> ("单组电压不均衡"=w2230:dbl)
                    n916 = call "输入分辨率计算-EV05.vi"("1字节?"=FALSE, "数值"=w2230, "偏移量"=0.0, "分辨率"=0.001) -> ("低字节"=w2232:dbl, "高字节1"=w2234:dbl)  [unwired: 1 in, 5 out]
                  }
                  frame Enabled {
                    w2237 = 255 ("高字节1")
                  }
                }
                n917 = Build Array(w2229, w2227) -> (w2228:i32[])
              }
              frame 6 {
                # "整组电压不均衡"
                n918 = disable-structure shown="启用" {
                  disable-tunnel: [w2246 w2249] -> w2241
                  disable-tunnel: [w2244 w2249] -> w2239
                  disable-tunnel: w2238 -> [w2243 _]
                  frame Disabled {
                    n919 = Unbundle By Name(w2243) -> ("整组电压不均衡"=w2242:dbl)
                    n920 = call "输入分辨率计算-EV05.vi"("1字节?"=FALSE, "数值"=w2242, "偏移量"=0.0, "分辨率"=0.001) -> ("低字节"=w2244:dbl, "高字节1"=w2246:dbl)  [unwired: 1 in, 5 out]
                  }
                  frame Enabled {
                    w2249 = 255 ("高字节1")
                  }
                }
                n921 = Build Array(w2241, w2239) -> (w2240:i32[])
              }
              frame 7 {
                # "单体电压过高"
                n922 = disable-structure shown="启用" {
                  disable-tunnel: [w2258 w2261] -> w2253
                  disable-tunnel: [w2256 w2261] -> w2251
                  disable-tunnel: w2250 -> [w2255 _]
                  frame Disabled {
                    n923 = Unbundle By Name(w2255) -> ("单体电压过高"=w2254:dbl)
                    n924 = call "输入分辨率计算-EV05.vi"("1字节?"=FALSE, "数值"=w2254, "偏移量"=0.0, "分辨率"=0.001) -> ("低字节"=w2256:dbl, "高字节1"=w2258:dbl)  [unwired: 1 in, 5 out]
                  }
                  frame Enabled {
                    w2261 = 255 ("高字节1")
                  }
                }
                n925 = Build Array(w2253, w2251) -> (w2252:i32[])
              }
              frame 8 {
                # "单体电压过低"
                n926 = disable-structure shown="启用" {
                  disable-tunnel: [w2270 w2273] -> w2265
                  disable-tunnel: [w2268 w2273] -> w2263
                  disable-tunnel: w2262 -> [w2267 _]
                  frame Disabled {
                    n927 = Unbundle By Name(w2267) -> ("单体电压过低"=w2266:dbl)
                    n928 = call "输入分辨率计算-EV05.vi"("1字节?"=FALSE, "数值"=w2266, "偏移量"=0.0, "分辨率"=0.001) -> ("低字节"=w2268:dbl, "高字节1"=w2270:dbl)  [unwired: 1 in, 5 out]
                  }
                  frame Enabled {
                    w2273 = 255 ("高字节1")
                  }
                }
                n929 = Build Array(w2265, w2263) -> (w2264:i32[])
              }
              frame 9 {
                # "充电电流过高"
                n930 = disable-structure shown="启用" {
                  disable-tunnel: [w2282 w2285] -> w2277
                  disable-tunnel: [w2280 w2285] -> w2275
                  disable-tunnel: w2274 -> [w2279 _]
                  frame Disabled {
                    n931 = Unbundle By Name(w2279) -> ("充电电流过高"=w2278:dbl)
                    n932 = call "输入分辨率计算-EV05.vi"("1字节?"=FALSE, "数值"=w2278, "偏移量"=-3000.0, "分辨率"=0.1) -> ("低字节"=w2280:dbl, "高字节1"=w2282:dbl)  [unwired: 1 in, 5 out]
                  }
                  frame Enabled {
                    w2285 = 255 ("高字节1")
                  }
                }
                n933 = Build Array(w2277, w2275) -> (w2276:i32[])
              }
              frame 10 {
                # "放电电流过高"
                n934 = disable-structure shown="启用" {
                  disable-tunnel: [w2294 w2297] -> w2289
                  disable-tunnel: [w2292 w2297] -> w2287
                  disable-tunnel: w2286 -> [w2291 _]
                  frame Disabled {
                    n935 = Unbundle By Name(w2291) -> ("放电电流过高"=w2290:dbl)
                    n936 = call "输入分辨率计算-EV05.vi"("1字节?"=FALSE, "数值"=w2290, "偏移量"=-3000.0, "分辨率"=0.1) -> ("低字节"=w2292:dbl, "高字节1"=w2294:dbl)  [unwired: 1 in, 5 out]
                  }
                  frame Enabled {
                    w2297 = 255 ("高字节1")
                  }
                }
                n937 = Build Array(w2289, w2287) -> (w2288:i32[])
              }
              frame 11 {
                # "单组温度不均衡"
                n938 = disable-structure shown="启用" {
                  disable-tunnel: [w2304 255 ("高字节1")] -> w2300
                  disable-tunnel: w2298 -> [w2302 _]
                  frame Disabled {
                    n939 = Unbundle By Name(w2302) -> ("单组温度不均衡"=w2301:dbl)
                    n940 = call "输入分辨率计算-EV05.vi"("1字节?"=TRUE, "数值"=w2301, "偏移量"=0.0, "分辨率"=1.0) -> ("高字节1"=w2304:dbl)  [unwired: 1 in, 6 out]
                  }
                  frame Enabled {
                  }
                }
                n941 = Build Array(w2300) -> (w2299:i32[])
              }
              frame 12 {
                # "SOC过高"
                n942 = Unbundle By Name(w2312) -> ("SOC过高"=w2311:dbl)
                n943 = call "输入分辨率计算-EV05.vi"("1字节?"=FALSE, "数值"=w2311, "偏移量"=0.0, "分辨率"=0.1) -> ("低字节"=w2313:dbl, "高字节1"=w2314:dbl)  [unwired: 1 in, 5 out]
                n944 = call "二进制解析-8.6.vi"("索引"=4, "数值"=w2314) -> ("低位子数组"=w2317:i32[])  [unwired: 3 out]
                n945 = call "二进制解析-8.6.vi"("索引"=4, "数值"=w2313) -> ("低位子数组"=w2309:i32[], "高位子数组"=w2316:i32[])  [unwired: 2 out]
                n946 = Insert Into Array(array=w2317, new element=w2316) -> (w2315:i32[])  [unwired: 1 in]
                n947 = call "数值二进制转十进制-8.6.vi"("子数组"=w2315) -> ("十进制数值"=w2310:i32)  [unwired: 4 out]
                n948 = disable-structure shown="启用" {
                  disable-tunnel: w2310 -> [w2325 _]
                  disable-tunnel: [w2325 255 ("高字节1")] -> w2308
                  disable-tunnel: [w2324 i32[] [] ("低位子数组 20")] -> _
                  disable-tunnel: w2309 -> [w2324 _]
                  frame Disabled {
                  }
                  frame Enabled {
                  }
                }
                n949 = Build Array(w2308, w2308) -> (w2321:i32[])
              }
              frame 13 {
                # "SOC过低"
                n950 = Unbundle By Name(w2334) -> ("SOC过低"=w2333:dbl)
                n951 = call "输入分辨率计算-EV05.vi"("1字节?"=FALSE, "数值"=w2333, "偏移量"=0.0, "分辨率"=0.1) -> ("低字节"=w2331:dbl, "高字节1"=w2332:dbl)  [unwired: 1 in, 5 out]
                n952 = call "二进制解析-8.6.vi"("索引"=4, "数值"=w2332) -> ("低位子数组"=w2329:i32[])  [unwired: 3 out]
                n953 = disable-structure shown="启用" {
                  disable-tunnel: w2331 -> [w2341 _]
                  disable-tunnel: [w2341 255 ("高字节1")] -> w2330
                  disable-tunnel: w2329 -> [w2340 _]
                  disable-tunnel: [_ 255 ("高字节1")] -> w2328
                  frame Disabled {
                    (unwired) i32[] [] ("低位子数组 4")
                  }
                  frame Enabled {
                  }
                }
                n954 = Build Array(w2328, w2330) -> (w2337:i32[])
              }
              frame 14 {
                # "内阻过大"
                n955 = disable-structure shown="启用" {
                  disable-tunnel: w2346 -> [w2351 _]
                  disable-tunnel: [w2347 255 ("高字节1")] -> w2344
                  frame Disabled {
                    n956 = Unbundle By Name(w2351) -> ("内阻过大"=w2350:dbl)
                    n957 = call "输入分辨率计算-EV05.vi"("1字节?"=TRUE, "数值"=w2350, "分辨率"=0.1) -> ("高字节1"=w2347:dbl)  [unwired: 2 in, 6 out]
                  }
                  frame Enabled {
                  }
                }
                n958 = Build Array(w2344) -> (w2345:i32[])
              }
              frame 15 {
                # "极柱温度过高"
                n959 = disable-structure shown="启用" {
                  disable-tunnel: w2355 -> [w2361 _]
                  disable-tunnel: [w2357 255 ("高字节1")] -> w2353
                  frame Disabled {
                    n960 = Unbundle By Name(w2361) -> ("极柱温度过高"=w2360:dbl)
                    n961 = call "输入分辨率计算-EV05.vi"("1字节?"=TRUE, "数值"=w2360, "偏移量"=-40.0, "分辨率"=1.0) -> ("高字节1"=w2357:dbl)  [unwired: 1 in, 6 out]
                  }
                  frame Enabled {
                  }
                }
                n962 = Build Array(w2353) -> (w2354:i32[])
              }
              frame 16 {
                # "SOH过低"
                n963 = disable-structure shown="启用" {
                  disable-tunnel: [w2378 w2386] -> w2365
                  disable-tunnel: w2364 -> [w2375 _]
                  disable-tunnel: [w2367 w2386] -> w2363
                  frame Disabled {
                    n964 = Unbundle By Name(w2375) -> ("SOH过低"=w2374:dbl)
                    n965 = call "输入分辨率计算-EV05.vi"("1字节?"=FALSE, "数值"=w2374, "偏移量"=0.0, "分辨率"=0.1) -> ("低字节"=w2376:dbl, "高字节1"=w2377:dbl)  [unwired: 1 in, 5 out]
                    n966 = call "二进制解析-8.6.vi"("索引"=4, "数值"=w2377) -> ("低位子数组"=w2380:i32[])  [unwired: 3 out]
                    n967 = call "二进制解析-8.6.vi"("索引"=4, "数值"=w2376) -> ("低位子数组"=w2369:i32[], "高位子数组"=w2379:i32[])  [unwired: 2 out]
                    n968 = call "二进制解析-8.6.vi"("索引"=4, "数值"=0) -> ("低位子数组"=w2370:i32[])  [unwired: 3 out]
                    n969 = Insert Into Array(array=w2380, new element=w2379) -> (w2373:i32[])  [unwired: 1 in]
                    n970 = Insert Into Array(array=w2369, new element=w2370) -> (w2368:i32[])  [unwired: 1 in]
                    n971 = call "数值二进制转十进制-8.6.vi"("子数组"=w2373) -> ("十进制数值"=w2378:i32)  [unwired: 4 out]
                    n972 = call "数值二进制转十进制-8.6.vi"("子数组"=w2368) -> ("十进制数值"=w2367:i32)  [unwired: 4 out]
                  }
                  frame Enabled {
                    w2386 = 255 ("高字节1")
                  }
                }
                n973 = Build Array(w2365, w2363) -> (w2366:i32[])
              }
            }
            n974 = Insert Into Array(array=w2170, new element=w2171) -> (w2169:dbl[])  [unwired: 1 in]
          }
          n975 = Build Array(w2166) -> (w2165:dbl[][])
          n976 = Build Array("二级故障阀值") -> (w2156:string[])
        }
        frame "总电压过高(3)" {
          n977 = Unbundle By Name(w2392) -> ("一级故障 3"=w2393:refnum<vi>)
          n978 = property class="Clust (严格)"(reference=w2393) -> ("Value"=w2391:T4)  [unwired: 1 in, 2 out]
          n979 = for {
            N: 17 -> [_]
            tunnel: w2391 -> [w2403]
            shift-right: [w2400] -> w2397
            shift-left: dbl[] [] -> [w2401]
            i -> [w2404]
            n980 = case shown="13" w2404 {
              tunnel: w2403 -> [w2405 w2416 w2427 w2437 w2447 w2457 w2469 w2481 w2493 w2505 w2517 w2529 w2543 w2565 w2577 w2586 w2595]
              tunnel: [w2406 w2417 w2428 w2438 w2448 w2459 w2471 w2483 w2495 w2507 w2519 w2530 w2552 w2568 w2576 w2585 w2597] -> w2402
              frame 0, Default {
                # "总电压过高"
                n981 = disable-structure shown="启用" {
                  disable-tunnel: [w2412 w2415] -> w2408
                  disable-tunnel: [w2411 w2415] -> w2407
                  disable-tunnel: w2405 -> [w2410 _]
                  frame Enabled {
                    n982 = Unbundle By Name(w2410) -> ("总电压过高"=w2409:dbl)
                    n983 = call "输入分辨率计算-EV05.vi"("1字节?"=FALSE, "数值"=w2409, "分辨率"=0.1) -> ("低字节"=w2412:dbl, "高字节1"=w2411:dbl)  [unwired: 2 in, 5 out]
                  }
                  frame Disabled {
                    w2415 = 255 ("高字节1")
                  }
                }
                n984 = Build Array(w2407, w2408) -> (w2406:dbl[])
              }
              frame 1 {
                # "总电压过低"
                n985 = disable-structure shown="启用" {
                  disable-tunnel: [w2423 w2426] -> w2419
                  disable-tunnel: [w2422 w2426] -> w2418
                  disable-tunnel: w2416 -> [w2421 _]
                  frame Disabled {
                    n986 = Unbundle By Name(w2421) -> ("总电压过低"=w2420:dbl)
                    n987 = call "输入分辨率计算-EV05.vi"("1字节?"=FALSE, "数值"=w2420, "分辨率"=0.1) -> ("低字节"=w2423:dbl, "高字节1"=w2422:dbl)  [unwired: 2 in, 5 out]
                  }
                  frame Enabled {
                    w2426 = 255 ("高字节1")
                  }
                }
                n988 = Build Array(w2418, w2419) -> (w2417:i32[])
              }
              frame 2 {
                # "温度过高"
                n989 = disable-structure shown="启用" {
                  disable-tunnel: [w2433 255 ("高字节1")] -> w2429
                  disable-tunnel: w2427 -> [w2431 _]
                  frame Disabled {
                    n990 = Unbundle By Name(w2431) -> ("温度过高"=w2430:dbl)
                    n991 = call "输入分辨率计算-EV05.vi"("1字节?"=TRUE, "数值"=w2430, "偏移量"=-40.0, "分辨率"=1.0) -> ("高字节1"=w2433:dbl)  [unwired: 1 in, 6 out]
                  }
                  frame Enabled {
                  }
                }
                n992 = Build Array(w2429) -> (w2428:i32[])
              }
              frame 3 {
                # "温度过低"
                n993 = disable-structure shown="启用" {
                  disable-tunnel: [w2443 255 ("高字节1")] -> w2439
                  disable-tunnel: w2437 -> [w2441 _]
                  frame Disabled {
                    n994 = Unbundle By Name(w2441) -> ("温度过低"=w2440:dbl)
                    n995 = call "输入分辨率计算-EV05.vi"("1字节?"=TRUE, "数值"=w2440, "偏移量"=-40.0, "分辨率"=1.0) -> ("高字节1"=w2443:dbl)  [unwired: 1 in, 6 out]
                  }
                  frame Enabled {
                  }
                }
                n996 = Build Array(w2439) -> (w2438:i32[])
              }
              frame 4 {
                # "整组温度不均衡"
                n997 = disable-structure shown="启用" {
                  disable-tunnel: [w2453 255 ("高字节1")] -> w2449
                  disable-tunnel: w2447 -> [w2451 _]
                  frame Disabled {
